vi "FGV FID THC Kalibrieren.vi"(8 "GT?":bool, 10 "Aktionen FID kalibrieren":T1, 11 "Sprachliste":string[][](array[string])) -> (1 "Zustand":string, 2 "Aktionen FID kalibrieren":T1)   [LabVIEW 2020, in "Auto Kalibrieren.lvlib"]
uses:
  Auto Kalibrieren.lvlib
  Aktionen FID kalibrieren.ctl
  Analysator Definition/FGV Analysator Definition Aktionen.ctl
  Seiten/CalGas Aufschaltung/FGV CalGas Aktionen.ctl
  Aktionen FGV Zustand Kalibrierung.ctl
  Aktion FGV CalZustand.ctl
  Seiten/EL3000/FID/Aktion FGV Messwerte_F.ctl
  Aktionen FGV AutoKAL Daten.ctl
  Seiten/EL3000/Allgemeine VI/FGV Uras26 Aktion.ctl
  Seiten/EL3000/FID/FID Kalibrierung/FID Kalibrieren.ctl
  Seiten/EL3000/Allgemeine VI/Allgemeine VI.lvlib
  Seiten/EL3000/FID/FID.lvlib
  Seiten/EL3000/FID/FID Kalibrierung/FID Kalibrierung.lvlib
  Analysator Definition/Analysator Definition.lvlib
  Seiten/CalGas Aufschaltung/CalGas Aufschaltung.lvlib
  Linearisierung V2/Linearisierung v2.lvlib
  Sprachverwaltung/Sprachverwaltung.lvlib
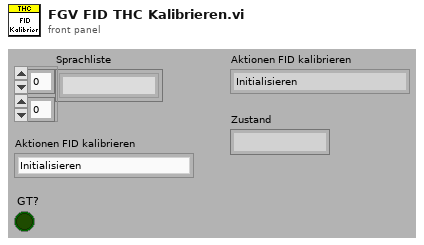
[diagram p1: front panel]
types:
  T1 = typedef "Auto Kalibrieren.lvlib/Aktionen FID kalibrieren.ctl" = enum16{"Initialisieren", "Warten auf FTIR", "Anstehende Störung", "0-Gas Aufschalten", "Nullpunkt Anfordern", "Nullpunkt", "Warten auf andere Messgeräte", "Messgas Aufschalten", "Endpunkt Anfordern", "Endpunkt", "Endpunkt kopieren", "Fertig", "Speichern"}
  T2 = typedef "Analysator Definition.lvlib/FGV Analysator Definition Aktionen.ctl" = enum16{"lesen", "MB setzen", "MB KAL setzen", "laden"}
  T3 = typedef "CalGas Aufschaltung.lvlib/FGV CalGas Aktionen.ctl" = enum16{"lesen", "Analysator Auswahl", "Def.CalGas", "Aufschaltung CalGas", "laden", "speichern", "KAL extrahieren"}
  T4 = typedef "Auto Kalibrieren.lvlib/Aktion FGV CalZustand.ctl" = enum16{"lesen", "Cal FTIR", "Cal FID CH4", "Cal PMA", "init", "Cal FID THC", "THC CG Eingang"}
  T5 = typedef "Auto Kalibrieren.lvlib/Aktionen FGV Zustand Kalibrierung.ctl" = enum16{"lesen", "LÖSCHEN", "Hintergrund fertig", "Nullpunkt NDIR CO lo", "Endpunkt NDIR CO lo", "Nullpunkt NDIR CO hi", "Endpunkt NDIR CO hi", "Nullpunkt NDIR CO2 lo", "Endpunkt NDIR CO2 lo", "Nullpunkt FID CH4", "Endpunkt FID CH4", "Nullpunkt FID THC", "Endpunkt FID THC", "Nullpunkt PMA", "Endpunkt PMA", "Fehler FT-IR", "Fehler NDIR lo", "Fehler FID CH4", "Fehler FID THC", "Fehler PMA", "TIMEOUT"}
  T6 = typedef "ABB-EL3000.lvlib/FID.lvlib/Aktion FGV Messwerte_F.ctl" = enum16{"lesen", "Messwerte", "Messbereich", "Status", "Diagnose Werte"}
  T7 = typedef "Auto Kalibrieren.lvlib/Aktionen FGV AutoKAL Daten.ctl" = enum16{"lesen", "laden", "speichern", "Aufschaltzeit"}
  T8 = typedef "ABB-EL3000.lvlib/FID.lvlib/FID Kalibrierung.lvlib/FID Kalibrieren.ctl" = enum16{"CH4 Nullpunkt", "THC Nullpunkt", "NMHC Nullpunkt", "CH4 Endpunkt", "THC Endpunkt", "NMHC Endpunkt"}
  T9 = typedef "ABB-EL3000.lvlib/Allgemeine VI.lvlib/FGV Uras26 Aktion.ctl" = enum16{"lesen", "CAL-Daten laden", "Messen", "Kalibrieren vorbereiten", "Kalibrieren", "CAL-Daten speichern", "Toleranz schreiben", "CAL-Daten kopieren"}
  T10 = typedef "Analysator Definition.lvlib/Betriebsdaten Komponente.ctl" = cluster{"Namen":string[], "MB Namen":string[], "Einheit":string, "MB Aktuell":u16, "MB Endwert":u16, "CalGase":u16[], "MB für KAL":u16[], "CG für KAL":u16[]}
  T11 = typedef "CalGas Aufschaltung.lvlib/Aufschaltung CalGas.ctl" = cluster{"Kalibriergas":T12, "Aufschaltpunkt":T13, "Analysator":T14}
  T12 = typedef "Auswahlfeld.ctl" = u16
  T13 = typedef "CalGas Aufschaltung.lvlib/Auswahl Aufschaltpunkt.ctl" = enum16{"über Filterblock", "Analysator direkt", "über PNS", "Entnahme", "Gasdivider"}
  T14 = typedef "CalGas Aufschaltung.lvlib/Auswahl Analysator.ctl" = enum16{"FT-IR", "FID", "PMA", "PMA/FID/FT-IR"}
  T15 = typedef "Auto Kalibrieren.lvlib/Zustand Messgeraete Kalibrierung.ctl" = cluster{"Hintergrund FT-IR":bool, "Nullpunkt NDIR CO lo":bool, "Endpunkt NDIR CO lo":bool, "Nullpunkt NDIR CO hi":bool, "Endpunkt NDIR CO hi":bool, "Nullpunkt NDIR CO2 lo":bool, "Endpunkt NDIR CO2 lo":bool, "Nullpunkt FID CH4":bool, "Endpunkt FID CH4":bool, "Nullpunkt FID THC":bool, "Endpunkt FID THC":bool, "Nullpunkt PMA":bool, "Endpunkt PMA":bool, "Fehler FT-IR":bool, "Fehler NDIR lo":bool, "Fehler FID CH4":bool, "Fehler FID THC":bool, "Fehler PMA":bool}
  T16 = cluster{"Ausfall":bool, "Funktionskontrolle":bool, "Wartungsbedarf":bool}
  T17 = typedef "Auto Kalibrieren.lvlib/Auschaltzeiten Null Endpunktgase.ctl" = cluster{"CO lo 0":sgl, "CO lo E":sgl, "CO hi 0":sgl, "CO hi E":sgl, "CO2 lo 0":sgl, "CO2 lo E":sgl, "CH4 0":sgl, "CH4 E":sgl, "THC 0":sgl, "THC E":sgl, "O2 0":sgl, "O2 E":sgl}
  T18 = typedef "String - Ausgabefeld.ctl" = string
  T19 = typedef "Zahlen-Ausgabefeld.ctl" = sgl
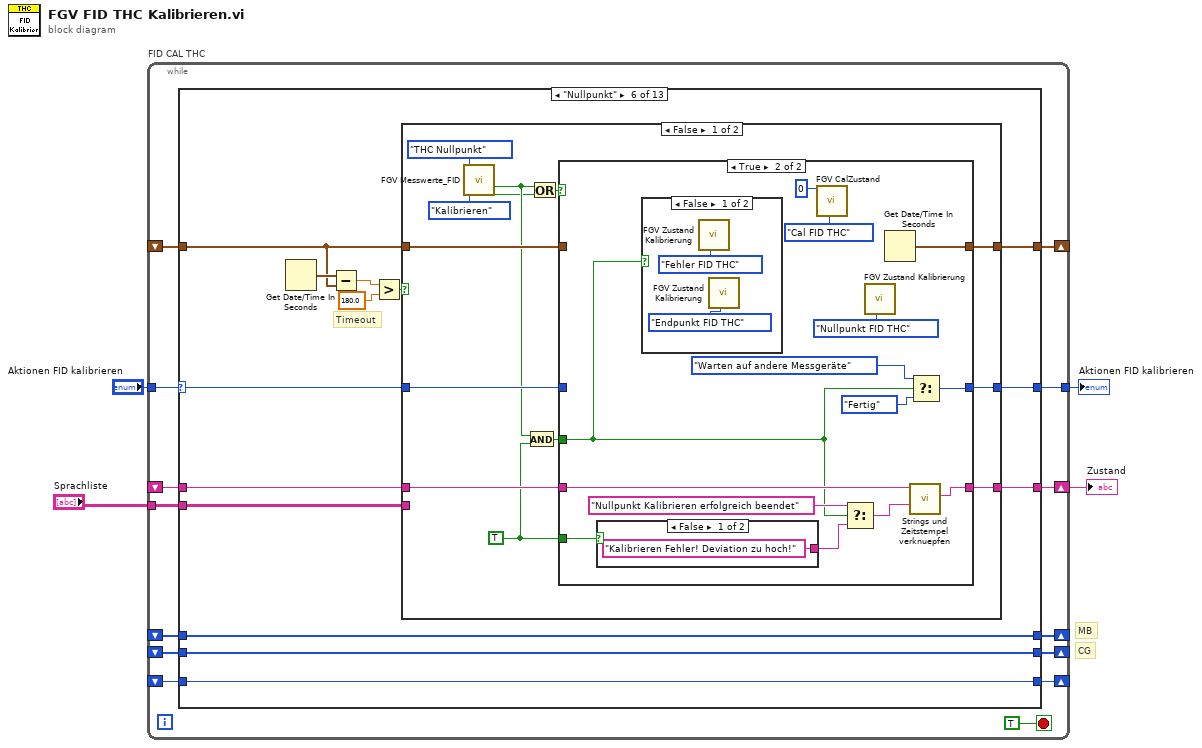
[diagram p0: block diagram]
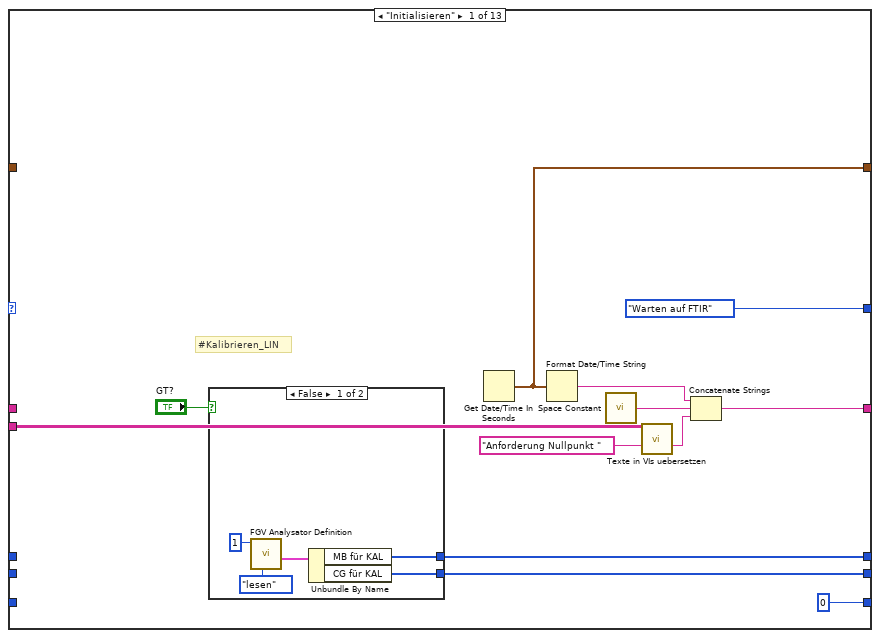
[diagram p2: hidden frame]
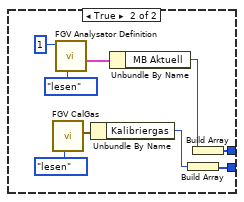
[diagram p3: hidden frame]
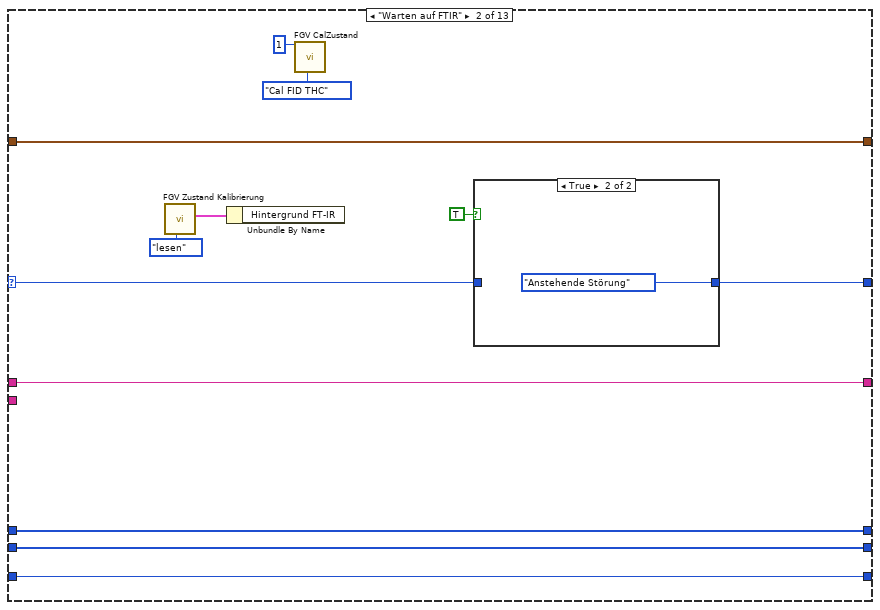
[diagram p4: hidden frame]
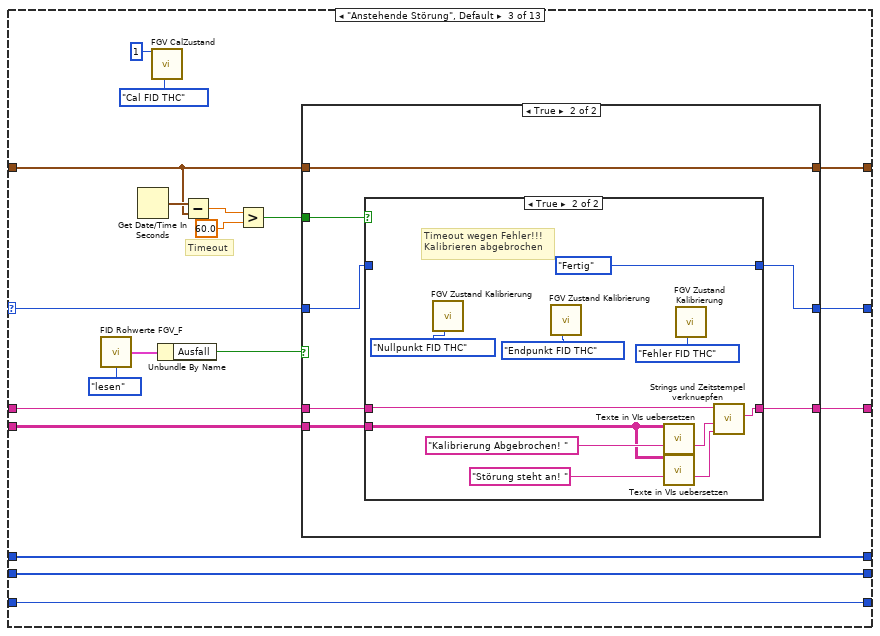
[diagram p6: hidden frame]
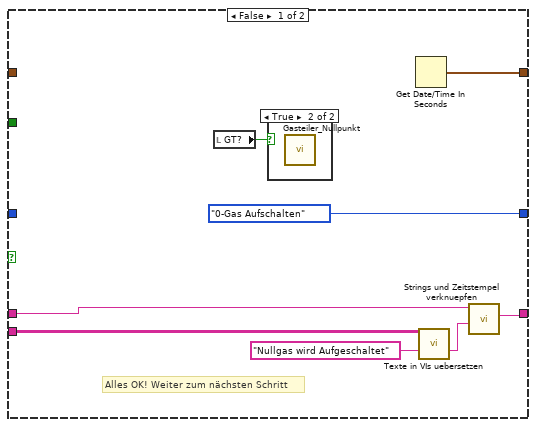
[diagram p7: hidden frame]
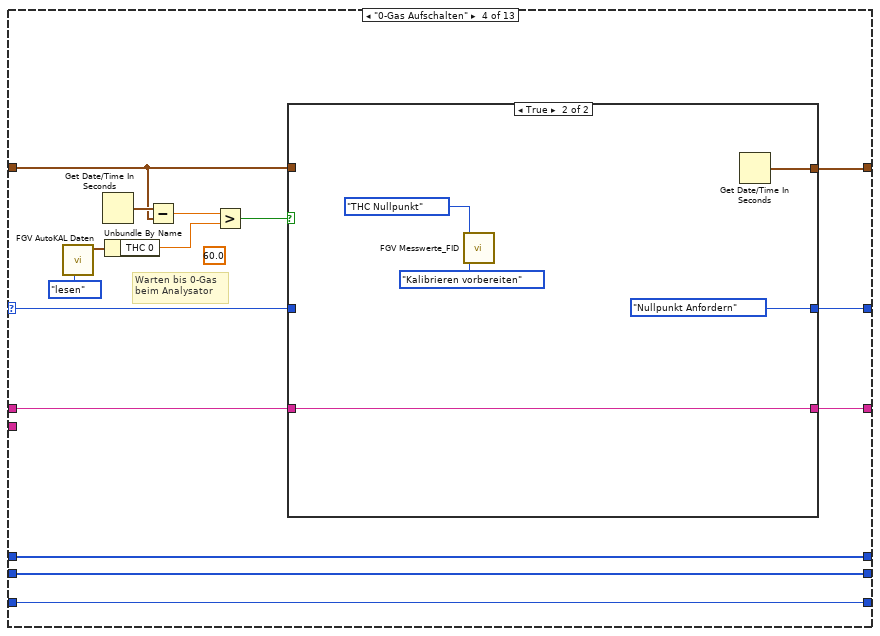
[diagram p10: hidden frame]
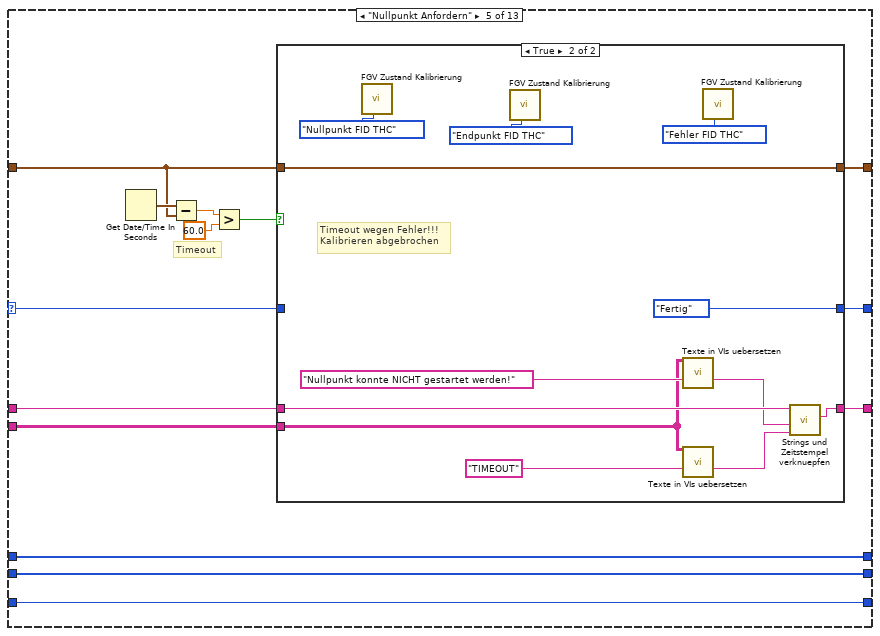
[diagram p12: hidden frame]
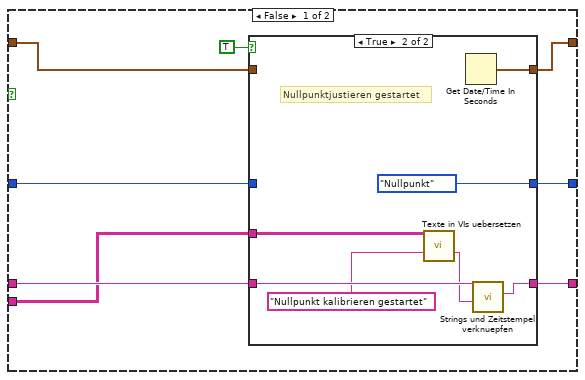
[diagram p13: hidden frame]
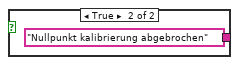
[diagram p16: hidden frame]
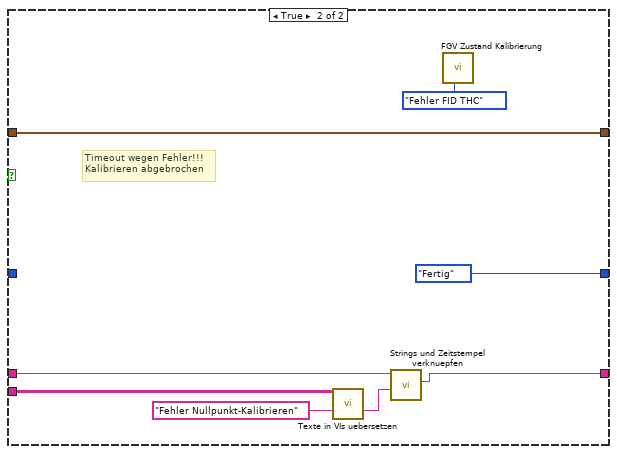
[diagram p18: hidden frame]
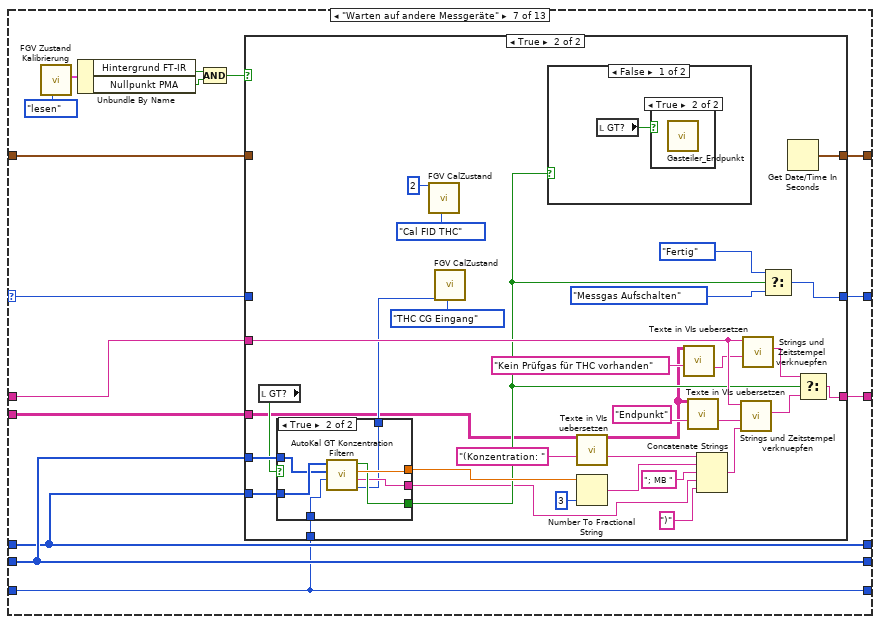
[diagram p19: hidden frame]
diagram:
  # "CG"
  # "MB"
  n1 = while "FID CAL THC" {
    shift-right: [w14] -> w4
    shift-left: _ -> [w16]
    shift-right: [w15] -> _
    shift-left: _ -> [w17]
    tunnel: "Aktionen FID kalibrieren" -> [w18]
    tunnel: [w13] -> w2
    shift-right: [w10] -> _
    shift-left: _ -> [w8]
    shift-right: [w11] -> _
    shift-left: _ -> [w9]
    shift-right: [w7] -> _
    shift-left: _ -> [w6]
    tunnel: "Sprachliste" -> [w5]
    stop <- TRUE stop-if-true
    n2 = case shown="\"Nullpunkt\"" w18 {
      selector: w18 -> [_ w51 w70 w115 w133 w177 w238 w306 w354 w401 _ w485 _]
      tunnel: w17 -> [_ w52 w68 w117 w138 w179 w239 w309 w359 w403 w461 w486 _]
      tunnel: w16 -> [_ w56 w73 w113 w135 w181 w241 w304 w356 w402 w453 w484 w500]
      tunnel: [w28 w52 w74 w116 w137 w178 w242 w308 w358 w400 w461 w486 w501] -> w15
      tunnel: [w27 w56 w72 w112 w134 w180 w240 w303 w355 w398 w451 w484 w500] -> w14
      tunnel: [Aktionen_FID_kalibrieren."Warten auf FTIR" ("Aktionen FID kalibrieren") w55 w69 w114 w136 w182 w243 w305 w357 w399 w459 w485 Aktionen_FID_kalibrieren."Fertig" ("Aktionen FID kalibrieren")] -> w13
      tunnel: [w24 w48 w62 w108 w132 w176 w231 w298 w353 w395 w458 w483 w497] -> w11
      tunnel: [w23 w47 w61 w107 w131 w175 w232 w299 w352 w396 w460 w482 w496] -> w10
      tunnel: w9 -> [_ w48 w62 w108 w132 w176 w231 w298 w353 w395 w458 w483 w497]
      tunnel: w8 -> [_ w47 w61 w107 w131 w175 w232 w299 w352 w396 w460 w482 w496]
      tunnel: [0 ("Komponente") w45 w60 w106 w130 w174 w230 w297 w351 w394 w456 w479 w494] -> w7
      tunnel: w6 -> [_ w45 w60 w106 w130 w174 w230 w297 w351 w394 w457 w479 w494]
      tunnel: w5 -> [w19 _ w59 _ w129 w173 w229 w296 w350 w392 w450 _ _]
      frame "Initialisieren" {
        # "#Kalibrieren_LIN"
        n3 = case shown="False" "GT?" {
          tunnel: [w35 w36] -> w24
          tunnel: [w34 w41] -> w23
          frame False {
            n4 = call "FGV Analysator Definition.vi"("Aktionen"=FGV_Analysator_Definition_Aktionen."lesen", "Komponente"=1) -> ("Betriebsdaten Komponente"=w32:T10)  [unwired: 5 in, 4 out]
            n5 = Unbundle By Name(w32) -> ("MB für KAL"=w35:u16[], "CG für KAL"=w34:u16[])
          }
          frame True {
            n6 = call "FGV CalGas.vi"("Aktionen"=FGV_CalGas_Aktionen."lesen") -> ("Aufschaltung CalGas"=w43:T11)  [unwired: 6 in, 4 out]
            n7 = call "FGV Analysator Definition.vi"("Aktionen"=FGV_Analysator_Definition_Aktionen."lesen", "Komponente"=1) -> ("Betriebsdaten Komponente"=w40:T10)  [unwired: 5 in, 4 out]
            n8 = Unbundle By Name(w43) -> ("Kalibriergas"=w42:T12)
            n9 = Unbundle By Name(w40) -> ("MB Aktuell"=w37:u16)
            n10 = Build Array(w42) -> (w41:T12[])
            n11 = Build Array(w37) -> (w36:u16[])
          }
        }
        n12 = Get Date/Time In Seconds() -> (seconds since 1Jan1904=w28:timestamp)
        n13 = Format Date/Time String(seconds (now)=w28) -> (date/time string=w30:string)  [unwired: 2 in]
        n14 = call <vilib>:"Space Constant.vi"() -> ("String"=w29:string)
        n15 = call "Texte in VIs uebersetzen.vi"("Sprachliste"=w19, "String zum Übersetzen"="Anforderung Nullpunkt " ("String")) -> ("String zum Übersetzen"=w20:string)  [unwired: 9 in, 4 out]
        n16 = Concatenate Strings(w30, w29, w20) -> (w27:string)
      }
      frame "Warten auf FTIR" {
        n17 = call "FGV Zustand Kalibrierung.vi"("Aktionen"=Aktionen_FGV_Zustand_Kalibrierung."lesen" ("Enum")) -> ("Zustand Kalibrierung"=w53:T15)  [unwired: 9 in, 1 out]
        n18 = Unbundle By Name(w53) -> ()  [unwired: 1 out]
        n19 = call "FGV CalZustand.vi"("CAL Zustand"=u16 1 ("CAL Zustand FTIR"), "Aktion"=Aktion_FGV_CalZustand."Cal FID THC") -> ()  [unwired: 13 in, 5 out]
        n20 = case shown="True" TRUE {
          tunnel: [w57 Aktionen_FID_kalibrieren."Anstehende Störung" ("Aktionen FID kalibrieren")] -> w55
          tunnel: w51 -> [w57 _]
          frame False {
          }
          frame True {
          }
        }
      }
      frame "Anstehende Störung", Default {
        # "Timeout"
        n21 = call "FID Rohwerte FGV_F.vi"("Aktion"=Aktion_FGV_Messwerte_F."lesen") -> ("Status"=w66:T16)  [unwired: 11 in, 3 out]
        n22 = Get Date/Time In Seconds() -> (seconds since 1Jan1904=w77:timestamp)
        n23 = call "FGV CalZustand.vi"("CAL Zustand"=u16 1 ("CAL Zustand FTIR"), "Aktion"=Aktion_FGV_CalZustand."Cal FID THC") -> ()  [unwired: 13 in, 5 out]
        n24 = Unbundle By Name(w66) -> ("Ausfall"=w67:bool)
        n25 = Subtract(x=w77, y=w68) -> (x-y=w76:dbl)
        n26 = Greater?(x=w76, y=60.0) -> (0:w71:bool)
        n27 = case shown="True" w67 {
          tunnel: [w85 w89] -> w74
          tunnel: w73 -> [w84 w88]
          tunnel: [w83 w87] -> w72
          tunnel: w71 -> [_ w92]
          tunnel: w70 -> [_ w91]
          tunnel: [Aktionen_FID_kalibrieren."0-Gas Aufschalten" ("Aktionen FID kalibrieren") w90] -> w69
          tunnel: w68 -> [_ w89]
          tunnel: w59 -> [w78 w86]
          frame False {
            # "Alles OK! Weiter zum nächsten Schritt"
            n28 = local read "GT?"() -> (w81:bool)
            n29 = case shown="True" w81 {
              frame False {
              }
              frame True {
                n30 = call "Gasteiler_Nullpunkt.vi"() -> ()  [unwired: 12 in]
              }
            }
            n31 = Get Date/Time In Seconds() -> (seconds since 1Jan1904=w85:timestamp)
            n32 = call "Texte in VIs uebersetzen.vi"("Sprachliste"=w78, "String zum Übersetzen"="Nullgas wird Aufgeschaltet" ("String 1 hinzufügen")) -> ("String zum Übersetzen"=w79:string)  [unwired: 9 in, 4 out]
            n33 = call "Strings und Zeitstempel verknuepfen.vi"("String 1 hinzufügen"=w79, "Eingagns String"=w84) -> ("Verknüpfter String"=w83:string)  [unwired: 9 in]
          }
          frame True {
            n34 = case shown="True" w92 {
              tunnel: w91 -> [w94 _]
              tunnel: [w94 Aktionen_FID_kalibrieren."Fertig" ("Aktionen FID kalibrieren")] -> w90
              tunnel: w88 -> [w93 w105]
              tunnel: [w93 w104] -> w87
              tunnel: w86 -> [_ w95]
              frame False {
                # "Fehler steht an!!!!"
              }
              frame True {
                # "Timeout wegen Fehler!!! \nKalibrieren abgebrochen"
                n35 = call "FGV Zustand Kalibrierung.vi"("Aktionen"=Aktionen_FGV_Zustand_Kalibrierung."Nullpunkt FID THC" ("Enum")) -> ()  [unwired: 9 in, 2 out]
                n36 = call "FGV Zustand Kalibrierung.vi"("Aktionen"=Aktionen_FGV_Zustand_Kalibrierung."Endpunkt FID THC" ("Enum")) -> ()  [unwired: 9 in, 2 out]
                n37 = call "Texte in VIs uebersetzen.vi"("Sprachliste"=w95, "String zum Übersetzen"="Kalibrierung Abgebrochen! " ("String")) -> ("String zum Übersetzen"=w96:string)  [unwired: 9 in, 4 out]
                n38 = call "Texte in VIs uebersetzen.vi"("Sprachliste"=w95, "String zum Übersetzen"="Störung steht an! " ("String")) -> ("String zum Übersetzen"=w98:string)  [unwired: 9 in, 4 out]
                n39 = call "FGV Zustand Kalibrierung.vi"("Aktionen"=Aktionen_FGV_Zustand_Kalibrierung."Fehler FID THC" ("Enum")) -> ()  [unwired: 9 in, 2 out]
                n40 = call "Strings und Zeitstempel verknuepfen.vi"("String 2 hinzufügen"=w98, "String 1 hinzufügen"=w96, "Eingagns String"=w105) -> ("Verknüpfter String"=w104:string)  [unwired: 8 in]
              }
            }
          }
        }
      }
      frame "0-Gas Aufschalten" {
        (unwired) 60.0 ("y")
        # "Warten bis 0-Gas \nbeim Analysator"
        n41 = call "FGV AutoKAL Daten.vi"("Aktionen"=Aktionen_FGV_AutoKAL_Daten."lesen") -> ("Aufschaltzeiten"=w110:T17)  [unwired: 10 in]
        n42 = Get Date/Time In Seconds() -> (seconds since 1Jan1904=w120:timestamp)
        n43 = Unbundle By Name(w110) -> ("THC 0"=w109:sgl)
        n44 = Subtract(x=w120, y=w117) -> (x-y=w119:dbl)
        n45 = Greater?(x=w119, y=w109) -> (0:w118:bool)
        n46 = case shown="True" w118 {
          tunnel: w117 -> [w123 _]
          tunnel: [w123 w128] -> w116
          tunnel: w115 -> [w122 _]
          tunnel: [w122 Aktionen_FID_kalibrieren."Nullpunkt Anfordern" ("Aktionen FID kalibrieren")] -> w114
          tunnel: w113 -> [w121 w127]
          tunnel: [w121 w127] -> w112
          frame False {
          }
          frame True {
            n47 = call "FGV Messwerte_FID.vi"("Kalibrieren"=FID_Kalibrieren."THC Nullpunkt", "Aktion"=FGV_Uras26_Aktion."Kalibrieren vorbereiten") -> ()  [unwired: 18 in, 8 out]
            n48 = Get Date/Time In Seconds() -> (seconds since 1Jan1904=w128:timestamp)
          }
        }
      }
      frame "Nullpunkt Anfordern" {
        # "Timeout"
        n49 = Get Date/Time In Seconds() -> (seconds since 1Jan1904=w142:timestamp)
        n50 = Subtract(x=w142, y=w138) -> (x-y=w141:dbl)
        n51 = Greater?(x=w141, y=60.0) -> (0:w139:bool)
        n52 = case shown="True" w139 {
          tunnel: w138 -> [w146 w172]
          tunnel: [w145 w172] -> w137
          tunnel: [w148 Aktionen_FID_kalibrieren."Fertig" ("Aktionen FID kalibrieren")] -> w136
          tunnel: w135 -> [w150 w171]
          tunnel: [w149 w170] -> w134
          tunnel: w133 -> [w147 _]
          tunnel: w129 -> [w143 w161]
          frame False {
            n53 = case shown="True" TRUE {
              tunnel: w150 -> [w151 w160]
              tunnel: [w151 w159] -> w149
              tunnel: [w153 Aktionen_FID_kalibrieren."Nullpunkt" ("Aktionen FID kalibrieren")] -> w148
              tunnel: w147 -> [w153 _]
              tunnel: w146 -> [w152 _]
              tunnel: [w152 w158] -> w145
              tunnel: w143 -> [_ w154]
              frame False {
              }
              frame True {
                # "Nullpunktjustieren gestartet"
                n54 = call "Texte in VIs uebersetzen.vi"("Sprachliste"=w154, "String zum Übersetzen"="Nullpunkt kalibrieren gestartet" ("String 1 hinzufügen")) -> ("String zum Übersetzen"=w155:string)  [unwired: 9 in, 4 out]
                n55 = Get Date/Time In Seconds() -> (seconds since 1Jan1904=w158:timestamp)
                n56 = call "Strings und Zeitstempel verknuepfen.vi"("String 1 hinzufügen"=w155, "Eingagns String"=w160) -> ("Verknüpfter String"=w159:string)  [unwired: 9 in]
              }
            }
          }
          frame True {
            # "Timeout wegen Fehler!!! \nKalibrieren abgebrochen"
            n57 = call "FGV Zustand Kalibrierung.vi"("Aktionen"=Aktionen_FGV_Zustand_Kalibrierung."Nullpunkt FID THC" ("Enum")) -> ()  [unwired: 9 in, 2 out]
            n58 = call "FGV Zustand Kalibrierung.vi"("Aktionen"=Aktionen_FGV_Zustand_Kalibrierung."Endpunkt FID THC" ("Enum")) -> ()  [unwired: 9 in, 2 out]
            n59 = call "Texte in VIs uebersetzen.vi"("Sprachliste"=w161, "String zum Übersetzen"="Nullpunkt konnte NICHT gestartet werden!" ("String")) -> ("String zum Übersetzen"=w164:string)  [unwired: 9 in, 4 out]
            n60 = call "Texte in VIs uebersetzen.vi"("Sprachliste"=w161, "String zum Übersetzen"="TIMEOUT" ("String")) -> ("String zum Übersetzen"=w162:string)  [unwired: 9 in, 4 out]
            n61 = call "FGV Zustand Kalibrierung.vi"("Aktionen"=Aktionen_FGV_Zustand_Kalibrierung."Fehler FID THC" ("Enum")) -> ()  [unwired: 9 in, 2 out]
            n62 = call "Strings und Zeitstempel verknuepfen.vi"("String 2 hinzufügen"=w162, "String 1 hinzufügen"=w164, "Eingagns String"=w171) -> ("Verknüpfter String"=w170:string)  [unwired: 8 in]
          }
        }
      }
      frame "Nullpunkt" {
        # "Timeout"
        n63 = Get Date/Time In Seconds() -> (seconds since 1Jan1904=w186:timestamp)
        n64 = Subtract(x=w186, y=w179) -> (x-y=w185:dbl)
        n65 = Greater?(x=w185, y=180.0) -> (0:w183:bool)
        n66 = case shown="False" w183 {
          tunnel: [w196 Aktionen_FID_kalibrieren."Fertig" ("Aktionen FID kalibrieren")] -> w182
          tunnel: w181 -> [w195 w228]
          tunnel: [w194 w227] -> w180
          tunnel: w179 -> [w199 w226]
          tunnel: [w198 w226] -> w178
          tunnel: w177 -> [w197 _]
          tunnel: w173 -> [_ w222]
          frame False {
            w191 = TRUE
            n67 = call "FGV Messwerte_FID.vi"("Kalibrieren"=FID_Kalibrieren."THC Nullpunkt", "Aktion"=FGV_Uras26_Aktion."Kalibrieren") -> ("Kalibrieren erfolgreich"=w188:bool, "CAL TimeOut"=w187:bool)  [unwired: 18 in, 6 out]
            n68 = And(x=w188, y=w191) -> (x .and. y?=w192:bool)
            n69 = Or(x=w188, y=w187) -> (x .or. y?=w193:bool)
            n70 = case shown="True" w193 {
              tunnel: w199 -> [w202 _]
              tunnel: [w202 w210] -> w198
              tunnel: w197 -> [w201 _]
              tunnel: [w201 w211] -> w196
              tunnel: w195 -> [w200 w216]
              tunnel: [w200 w215] -> w194
              tunnel: w192 -> [_ w208]
              tunnel: w191 -> [_ w207]
              frame False {
              }
              frame True {
                n71 = case shown="False" w207 {
                  tunnel: ["Kalibrieren Fehler! Deviation zu hoch!" ("String 1 hinzufügen") "Nullpunkt kalibrierung abgebrochen" ("String 1 hinzufügen")] -> w213
                  frame False {
                  }
                  frame True {
                  }
                }
                n72 = case shown="False" w208 {
                  frame False {
                    n73 = call "FGV Zustand Kalibrierung.vi"("Aktionen"=Aktionen_FGV_Zustand_Kalibrierung."Fehler FID THC" ("Enum")) -> ()  [unwired: 9 in, 2 out]
                    n74 = call "FGV Zustand Kalibrierung.vi"("Aktionen"=Aktionen_FGV_Zustand_Kalibrierung."Endpunkt FID THC" ("Enum")) -> ()  [unwired: 9 in, 2 out]
                  }
                  frame True {
                  }
                }
                n75 = call "FGV CalZustand.vi"("CAL Zustand"=u16 0 ("CAL Zustand FTIR"), "Aktion"=Aktion_FGV_CalZustand."Cal FID THC") -> ()  [unwired: 13 in, 5 out]
                n76 = Select(t="Nullpunkt Kalibrieren erfolgreich beendet" ("String 1 hinzufügen"), s=w208, f=w213) -> (s? t:f=w212:string)
                n77 = call "FGV Zustand Kalibrierung.vi"("Aktionen"=Aktionen_FGV_Zustand_Kalibrierung."Nullpunkt FID THC" ("Enum")) -> ()  [unwired: 9 in, 2 out]
                n78 = Get Date/Time In Seconds() -> (seconds since 1Jan1904=w210:timestamp)
                n79 = call "Strings und Zeitstempel verknuepfen.vi"("String 1 hinzufügen"=w212, "Eingagns String"=w216) -> ("Verknüpfter String"=w215:string)  [unwired: 9 in]
                n80 = Select(t=Aktionen_FID_kalibrieren."Warten auf andere Messgeräte" ("Aktionen FID kalibrieren"), s=w208, f=Aktionen_FID_kalibrieren."Fertig" ("Aktionen FID kalibrieren")) -> (s? t:f=w211:T1)
              }
            }
          }
          frame True {
            # "Timeout wegen Fehler!!! \nKalibrieren abgebrochen"
            n81 = call "Texte in VIs uebersetzen.vi"("Sprachliste"=w222, "String zum Übersetzen"="Fehler Nullpunkt-Kalibrieren" ("String 1 hinzufügen")) -> ("String zum Übersetzen"=w223:string)  [unwired: 9 in, 4 out]
            n82 = call "Strings und Zeitstempel verknuepfen.vi"("String 1 hinzufügen"=w223, "Eingagns String"=w228) -> ("Verknüpfter String"=w227:string)  [unwired: 9 in]
            n83 = call "FGV Zustand Kalibrierung.vi"("Aktionen"=Aktionen_FGV_Zustand_Kalibrierung."Fehler FID THC" ("Enum")) -> ()  [unwired: 9 in, 2 out]
          }
        }
      }
      frame "Warten auf andere Messgeräte" {
        n84 = call "FGV Zustand Kalibrierung.vi"("Aktionen"=Aktionen_FGV_Zustand_Kalibrierung."lesen" ("Enum")) -> ("Zustand Kalibrierung"=w236:T15)  [unwired: 9 in, 1 out]
        n85 = Unbundle By Name(w236) -> ("Hintergrund FT-IR"=w235:bool, "Nullpunkt PMA"=w233:bool)
        n86 = Compound Arithmetic op=AND(w235, w233) -> (w234:bool)
        n87 = case shown="True" w234 {
          tunnel: [w245 w274] -> w243
          tunnel: [w246 w278] -> w242
          tunnel: w241 -> [w244 w276]
          tunnel: [w244 w275] -> w240
          tunnel: w239 -> [w246 _]
          tunnel: w238 -> [w245 _]
          tunnel: w232 -> [_ w264]
          tunnel: w231 -> [_ w263]
          tunnel: w230 -> [_ w259]
          tunnel: w229 -> [_ w248]
          frame False {
          }
          frame True {
            n88 = local read "GT?"() -> (w255:bool)
            n89 = case shown="True" w255 {
              tunnel: [w285 w293] -> w266
              tunnel: [w284 w292] -> w265
              tunnel: w264 -> [w283 w289]
              tunnel: w263 -> [w282 w290]
              tunnel: [w281 w291] -> w261
              tunnel: w259 -> [w280 w287]
              tunnel: [w279 w288] -> w256
              frame False {
                n90 = Index Array(array=w282, index=w280) -> (element=w286:u16)
                n91 = Index Array(array=w283, index=w280) -> (element=w279:T12)
                n92 = call "CalGas Filtern für Endpunktkalibrieren.vi"("Messbereich"=w286, "CalGas"=w279) -> ("Messberich"=w281:T18, "Wert 1"=w285:T19, "Fehler"=w284:bool)  [unwired: 2 in, 5 out]
              }
              frame True {
                n93 = call "AutoKal GT Konzentration Filtern.vi"("Index"=w287, "CG für KAL"=w289, "MB für KAL"=w290) -> ("CG für KAL"=w288:T12, "Messberich"=w291:T18, "Konzentration"=w293:dbl, "Fehler/Leer"=w292:bool)  [unwired: 5 in]
              }
            }
            n94 = call "FGV CalZustand.vi"("CAL Zustand"=u16 2, "Aktion"=Aktion_FGV_CalZustand."Cal FID THC") -> ()  [unwired: 13 in, 5 out]
            n95 = call "FGV CalZustand.vi"("CG Eingang"=w256, "Aktion"=Aktion_FGV_CalZustand."THC CG Eingang") -> ()  [unwired: 13 in, 5 out]
            n96 = case shown="False" w265 {
              frame False {
                n97 = local read "GT?"() -> (w294:bool)
                n98 = case shown="True" w294 {
                  frame False {
                  }
                  frame True {
                    n99 = call "Gasteiler_Endpunkt.vi"() -> ()  [unwired: 12 in]
                  }
                }
              }
              frame True {
                n100 = call "FGV Zustand Kalibrierung.vi"("Aktionen"=Aktionen_FGV_Zustand_Kalibrierung."Fehler FID THC" ("Enum")) -> ()  [unwired: 9 in, 2 out]
              }
            }
            n101 = call "Texte in VIs uebersetzen.vi"("Sprachliste"=w248, "String zum Übersetzen"="(Konzentration: " ("String")) -> ("Sprachliste out"=w247:string[][], "String zum Übersetzen"=w249:string)  [unwired: 9 in, 3 out]
            n102 = Number To Fractional String(number=w266, precision (6)=i16 3 ("Genauigkeit (6)")) -> (F-format string=w272:string)  [unwired: 2 in]
            n103 = call "Texte in VIs uebersetzen.vi"("Sprachliste"=w247, "String zum Übersetzen"="Kein Prüfgas für THC vorhanden" ("String 1 hinzufügen")) -> ("String zum Übersetzen"=w253:string)  [unwired: 9 in, 4 out]
            n104 = call "Texte in VIs uebersetzen.vi"("Sprachliste"=w247, "String zum Übersetzen"="Endpunkt" ("String 1 hinzufügen")) -> ("String zum Übersetzen"=w251:string)  [unwired: 9 in, 4 out]
            n105 = Concatenate Strings(w249, w272, "; MB " ("String"), w261, ")" ("String")) -> (w277:string)
            n106 = call "Strings und Zeitstempel verknuepfen.vi"("String 2 hinzufügen"=w277, "String 1 hinzufügen"=w251, "Eingagns String"=w276) -> ("Verknüpfter String"=w270:string)  [unwired: 8 in]
            n107 = call "Strings und Zeitstempel verknuepfen.vi"("String 1 hinzufügen"=w253, "Eingagns String"=w276) -> ("Verknüpfter String"=w271:string)  [unwired: 9 in]
            n108 = Select(t=Aktionen_FID_kalibrieren."Fertig" ("Aktionen FID kalibrieren"), s=w265, f=Aktionen_FID_kalibrieren."Messgas Aufschalten" ("Aktionen FID kalibrieren")) -> (s? t:f=w274:T1)
            n109 = Get Date/Time In Seconds() -> (seconds since 1Jan1904=w278:timestamp)
            n110 = Select(t=w271, s=w265, f=w270) -> (s? t:f=w275:string)
          }
        }
      }
      frame "Messgas Aufschalten" {
        (unwired) 60.0 ("y")
        # "Warten bis Endpunktgas\nbei Analysator"
        n111 = call "FGV AutoKAL Daten.vi"("Aktionen"=Aktionen_FGV_AutoKAL_Daten."lesen") -> ("Aufschaltzeiten"=w301:T17)  [unwired: 10 in]
        n112 = Unbundle By Name(w301) -> ("THC E"=w300:sgl)
        n113 = Get Date/Time In Seconds() -> (seconds since 1Jan1904=w311:timestamp)
        n114 = Subtract(x=w311, y=w309) -> (x-y=w310:dbl)
        n115 = Greater?(x=w310, y=w300) -> (0:w307:bool)
        n116 = case shown="True" w307 {
          tunnel: w309 -> [w314 _]
          tunnel: [w314 w331] -> w308
          tunnel: w306 -> [w313 _]
          tunnel: [w313 Aktionen_FID_kalibrieren."Endpunkt Anfordern" ("Aktionen FID kalibrieren")] -> w305
          tunnel: w304 -> [w312 w332]
          tunnel: [w312 w333] -> w303
          tunnel: w299 -> [_ w323]
          tunnel: w298 -> [_ w322]
          tunnel: w297 -> [_ w321]
          tunnel: w296 -> [_ w316]
          frame False {
          }
          frame True {
            n117 = local read "GT?"() -> (w324:bool)
            n118 = case shown="True" w324 {
              tunnel: [w342 w349] -> w325
              tunnel: [w341 w348] -> _
              tunnel: w323 -> [w340 w345]
              tunnel: w322 -> [w339 w346]
              tunnel: [w338 w347] -> _
              tunnel: w321 -> [w337 _]
              tunnel: [w336 w344] -> _
              frame False {
                n119 = Index Array(array=w339, index=w337) -> (element=w343:u16)
                n120 = Index Array(array=w340, index=w337) -> (element=w336:T12)
                n121 = call "CalGas Filtern für Endpunktkalibrieren.vi"("Messbereich"=w343, "CalGas"=w336) -> ("Messberich"=w338:T18, "Wert 1"=w342:T19, "Fehler"=w341:bool)  [unwired: 2 in, 5 out]
              }
              frame True {
                n122 = call "AutoKal GT Konzentration Filtern.vi"("CG für KAL"=w345, "MB für KAL"=w346) -> ("CG für KAL"=w344:T12, "Messberich"=w347:T18, "Konzentration"=w349:dbl, "Fehler/Leer"=w348:bool)  [unwired: 6 in]
              }
            }
            n123 = call "FGV Messwerte_FID.vi"("Prüfgaskonz."=w325, "Kalibrieren"=FID_Kalibrieren."THC Endpunkt", "Aktion"=FGV_Uras26_Aktion."Kalibrieren vorbereiten") -> ()  [unwired: 17 in, 8 out]
            n124 = call "Texte in VIs uebersetzen.vi"("Sprachliste"=w316, "String zum Übersetzen"="(Konzentration: " ("String")) -> ("Sprachliste out"=w315:string[][], "String zum Übersetzen"=w317:string)  [unwired: 9 in, 3 out]
            n125 = Number To Fractional String(number=w325, precision (6)=i16 1 ("Genauigkeit (6)")) -> (F-format string=w329:string)  [unwired: 2 in]
            n126 = call "Texte in VIs uebersetzen.vi"("Sprachliste"=w315, "String zum Übersetzen"="Anforderung Endpunkt kalibrieren" ("String 1 hinzufügen")) -> ("String zum Übersetzen"=w319:string)  [unwired: 9 in, 4 out]
            n127 = Concatenate Strings(w317, w329, ")" ("String")) -> (w334:string)
            n128 = Get Date/Time In Seconds() -> (seconds since 1Jan1904=w331:timestamp)
            n129 = call "Strings und Zeitstempel verknuepfen.vi"("String 2 hinzufügen"=w334, "String 1 hinzufügen"=w319, "Eingagns String"=w332) -> ("Verknüpfter String"=w333:string)  [unwired: 8 in]
          }
        }
      }
      frame "Endpunkt Anfordern" {
        # "Timeout"
        n130 = Get Date/Time In Seconds() -> (seconds since 1Jan1904=w363:timestamp)
        n131 = Subtract(x=w363, y=w359) -> (x-y=w362:dbl)
        n132 = Greater?(x=w362, y=100.0) -> (0:w360:bool)
        n133 = case shown="False" w360 {
          tunnel: w359 -> [w371 w391]
          tunnel: [w366 w391] -> w358
          tunnel: [w367 Aktionen_FID_kalibrieren."Fertig" ("Aktionen FID kalibrieren")] -> w357
          tunnel: w356 -> [w369 w390]
          tunnel: [w368 w389] -> w355
          tunnel: w354 -> [w370 _]
          tunnel: w350 -> [w364 w382]
          frame False {
            n134 = case shown="False" TRUE {
              tunnel: w369 -> [w372 w381]
              tunnel: [w372 w380] -> w368
              tunnel: [w374 Aktionen_FID_kalibrieren."Endpunkt" ("Aktionen FID kalibrieren")] -> w367
              tunnel: w370 -> [w374 _]
              tunnel: w371 -> [w373 _]
              tunnel: [w373 w379] -> w366
              tunnel: w364 -> [_ w375]
              frame False {
              }
              frame True {
                # "Endpunkt Kalibrieren gestartet"
                n135 = call "Texte in VIs uebersetzen.vi"("Sprachliste"=w375, "String zum Übersetzen"="Endpunkt kalibrieren gestartet" ("String 1 hinzufügen")) -> ("String zum Übersetzen"=w376:string)  [unwired: 9 in, 4 out]
                n136 = Get Date/Time In Seconds() -> (seconds since 1Jan1904=w379:timestamp)
                n137 = call "Strings und Zeitstempel verknuepfen.vi"("String 1 hinzufügen"=w376, "Eingagns String"=w381) -> ("Verknüpfter String"=w380:string)  [unwired: 9 in]
              }
            }
          }
          frame True {
            # "Timeout wegen Fehler!!! \nKalibrieren abgebrochen"
            n138 = call "FGV Zustand Kalibrierung.vi"("Aktionen"=Aktionen_FGV_Zustand_Kalibrierung."Fehler FID THC" ("Enum")) -> ()  [unwired: 9 in, 2 out]
            n139 = call "Texte in VIs uebersetzen.vi"("Sprachliste"=w382, "String zum Übersetzen"="TIMEOUT" ("String")) -> ("String zum Übersetzen"=w383:string)  [unwired: 9 in, 4 out]
            n140 = call "Texte in VIs uebersetzen.vi"("Sprachliste"=w382, "String zum Übersetzen"="Endpunkt konnte NICHT gestartet werden!" ("String")) -> ("String zum Übersetzen"=w385:string)  [unwired: 9 in, 4 out]
            n141 = call "Strings und Zeitstempel verknuepfen.vi"("String 2 hinzufügen"=w383, "String 1 hinzufügen"=w385, "Eingagns String"=w390) -> ("Verknüpfter String"=w389:string)  [unwired: 8 in]
          }
        }
      }
      frame "Endpunkt" {
        # "Timeout"
        n142 = Get Date/Time In Seconds() -> (seconds since 1Jan1904=w406:timestamp)
        n143 = Subtract(x=w406, y=w403) -> (x-y=w405:dbl)
        n144 = Greater?(x=w405, y=180.0) -> (0:w397:bool)
        n145 = Index Array(array=w395, index=w394) -> (element=w393:u16)
        n146 = case shown="False" w397 {
          tunnel: [w419 Aktionen_FID_kalibrieren."Fertig" ("Aktionen FID kalibrieren")] -> w399
          tunnel: w402 -> [w418 w449]
          tunnel: [w417 w448] -> w398
          tunnel: w403 -> [w422 w447]
          tunnel: [w421 w447] -> w400
          tunnel: w401 -> [w420 _]
          tunnel: w393 -> [w409 _]
          tunnel: w392 -> [w407 w442]
          frame False {
            w414 = TRUE
            n147 = Decrement(x=w409) -> (x-1=w408:u16)
            n148 = call "FGV Messwerte_FID.vi"("Messbereich"=w408, "Kalibrieren"=FID_Kalibrieren."THC Endpunkt", "Aktion"=FGV_Uras26_Aktion."Kalibrieren") -> ("Kalibrieren erfolgreich"=w411:bool, "CAL TimeOut"=w410:bool)  [unwired: 17 in, 6 out]
            n149 = Or(x=w411, y=w410) -> (x .or. y?=w416:bool)
            n150 = And(x=w411, y=w414) -> (x .and. y?=w415:bool)
            n151 = case shown="True" w416 {
              tunnel: w422 -> [w425 _]
              tunnel: [w425 w434] -> w421
              tunnel: w420 -> [w424 _]
              tunnel: [w424 w433] -> w419
              tunnel: w418 -> [w423 w438]
              tunnel: [w423 w437] -> w417
              tunnel: w415 -> [_ w432]
              tunnel: w414 -> [_ w431]
              tunnel: w407 -> [_ w426]
              frame False {
              }
              frame True {
                n152 = case shown="True" w431 {
                  tunnel: ["Kalibriern Fehler! Deviation zu Hoch!" ("String 1 hinzufügen") "Endpunkt Kalibrierung abgebrochen!" ("String 1 hinzufügen")] -> w435
                  frame False {
                  }
                  frame True {
                  }
                }
                n153 = case shown="False" w432 {
                  frame False {
                    n154 = call "FGV Zustand Kalibrierung.vi"("Aktionen"=Aktionen_FGV_Zustand_Kalibrierung."Fehler FID THC" ("Enum")) -> ()  [unwired: 9 in, 2 out]
                  }
                  frame True {
                  }
                }
                n155 = Select(t="Endpunkt Kalibrierung erfolgreich beendet" ("String 1 hinzufügen"), s=w432, f=w435) -> (s? t:f=w428:string)
                n156 = Get Date/Time In Seconds() -> (seconds since 1Jan1904=w434:timestamp)
                n157 = call "Texte in VIs uebersetzen.vi"("Sprachliste"=w426, "String zum Übersetzen"=w428) -> ("String zum Übersetzen"=w427:string)  [unwired: 9 in, 4 out]
                n158 = call "Strings und Zeitstempel verknuepfen.vi"("String 1 hinzufügen"=w427, "Eingagns String"=w438) -> ("Verknüpfter String"=w437:string)  [unwired: 9 in]
                n159 = Select(t=Aktionen_FID_kalibrieren."Endpunkt kopieren" ("Aktionen FID kalibrieren"), s=w432, f=Aktionen_FID_kalibrieren."Fertig" ("Aktionen FID kalibrieren")) -> (s? t:f=w433:T1)
              }
            }
          }
          frame True {
            # "Timeout wegen Fehler!!! \nKalibrieren abgebrochen"
            n160 = call "FGV Zustand Kalibrierung.vi"("Aktionen"=Aktionen_FGV_Zustand_Kalibrierung."Fehler FID THC" ("Enum")) -> ()  [unwired: 9 in, 2 out]
            n161 = call "Texte in VIs uebersetzen.vi"("Sprachliste"=w442, "String zum Übersetzen"="Fehler Endpunkt-Kalibrieren" ("String 1 hinzufügen")) -> ("String zum Übersetzen"=w443:string)  [unwired: 9 in, 4 out]
            n162 = call "Strings und Zeitstempel verknuepfen.vi"("String 1 hinzufügen"=w443, "Eingagns String"=w449) -> ("Verknüpfter String"=w448:string)  [unwired: 9 in]
          }
        }
      }
      frame "Endpunkt kopieren" {
        n163 = Increment(x=w457) -> (x+1=w456:i32)
        n164 = Index Array(array=w458, index=w456) -> (element=w454:u16)
        n165 = Greater Than 0?(x=w454) -> (x > 0?=w455:bool)
        n166 = case shown="True" w455 {
          tunnel: [Aktionen_FID_kalibrieren."Speichern" ("Aktionen FID kalibrieren") Aktionen_FID_kalibrieren."Warten auf andere Messgeräte" ("Aktionen FID kalibrieren")] -> w459
          tunnel: w454 -> [_ w476]
          tunnel: [w463 w474] -> w452
          tunnel: w450 -> [w462 w469]
          frame False {
            n167 = call "FGV Messwerte_FID.vi"("Kalibrieren"=FID_Kalibrieren."THC Endpunkt", "Aktion"=FGV_Uras26_Aktion."CAL-Daten kopieren") -> ()  [unwired: 18 in, 8 out]
            n168 = call "FGV Zustand Kalibrierung.vi"("Aktionen"=Aktionen_FGV_Zustand_Kalibrierung."Endpunkt FID THC" ("Enum")) -> ()  [unwired: 9 in, 2 out]
            n169 = call "Texte in VIs uebersetzen.vi"("Sprachliste"=w462, "String zum Übersetzen"="Endpunkte kopiert" ("String 1 hinzufügen")) -> ("String zum Übersetzen"=w463:string)  [unwired: 9 in, 4 out]
          }
          frame True {
            n170 = Number To Decimal String(number=w476) -> (decimal integer string=w475:string)  [unwired: 1 in]
            n171 = call "Texte in VIs uebersetzen.vi"("Sprachliste"=w469, "String zum Übersetzen"="Messbereich") -> ("String zum Übersetzen"=w472:string)  [unwired: 9 in, 4 out]
            n172 = call "Texte in VIs uebersetzen.vi"("Sprachliste"=w469, "String zum Übersetzen"="wird kalibriert.") -> ("String zum Übersetzen"=w470:string)  [unwired: 9 in, 4 out]
            n173 = Concatenate Strings(w472, w475, w470) -> (w474:string)
          }
        }
        n174 = call "Strings und Zeitstempel verknuepfen.vi"("String 1 hinzufügen"=w452, "Eingagns String"=w453) -> ("Verknüpfter String"=w451:string)  [unwired: 9 in]
      }
      frame "Fertig" {
        n175 = disable-structure shown="Deaktiviert" {
          frame Disabled {
            n176 = call "FGV Zustand Kalibrierung.vi"("Aktionen"=Aktionen_FGV_Zustand_Kalibrierung."lesen" ("Enum")) -> ("Zustand Kalibrierung"=w490:T15)  [unwired: 9 in, 1 out]
            n177 = Unbundle By Name(w490) -> ("Nullpunkt FID THC"=w489:bool, "Endpunkt FID THC"=w488:bool)
            n178 = And(x=w489, y=w488) -> (x .and. y?=w487:bool)
            n179 = case shown="True" w487 {
              frame False {
              }
              frame True {
                n180 = call "FGV CalZustand.vi"("CAL Zustand"=u16 0 ("CAL Zustand FTIR"), "Aktion"=Aktion_FGV_CalZustand."Cal FID THC") -> ()  [unwired: 13 in, 5 out]
              }
            }
          }
          frame Enabled {
          }
        }
        n181 = call "FGV CalZustand.vi"("CAL Zustand"=u16 0 ("CAL Zustand FTIR"), "Aktion"=Aktion_FGV_CalZustand."Cal FID THC") -> ()  [unwired: 13 in, 5 out]
        n182 = local read "GT?"() -> (w478:bool)
        n183 = case shown="True" w478 {
          frame False {
          }
          frame True {
            n184 = call "Gasteiler_Standby.vi"() -> ()  [unwired: 12 in]
          }
        }
      }
      frame "Speichern" {
        n185 = call "FGV Zustand Kalibrierung.vi"("Aktionen"=Aktionen_FGV_Zustand_Kalibrierung."Endpunkt FID THC" ("Enum")) -> ()  [unwired: 9 in, 2 out]
        n186 = call "FGV Messwerte_FID.vi"("Aktion"=FGV_Uras26_Aktion."CAL-Daten speichern") -> ()  [unwired: 19 in, 8 out]
        n187 = Get Date/Time In Seconds() -> (seconds since 1Jan1904=w501:timestamp)
      }
    }
  }
  "Zustand" <- w4
  "Aktionen FID kalibrieren" <- w2
